vi "Launch Client LNA.vi"(8 "error in (no error)":errorcluster, 11 "Client Controller in":refnum<class "Client Controller.lvclass">) -> (0 "error out":errorcluster, 3 "Client Controller out":refnum<class "Client Controller.lvclass">)   [LabVIEW 2016, in "Client Controller.lvlib" / "Client Controller.lvclass"]
uses:
  Client Controller.lvclass
  C:/Program Files (x86)/National Instruments/LabVIEW 2016/vi.lib/ActorFramework/Actor/Actor.lvclass
  Client LNA/Client LNA.lvclass
  C:/Program Files (x86)/National Instruments/LabVIEW 2016/vi.lib/NI/Actors/Linked Network Actor/Linked Network Actor/Linked Network Actor.lvclass
  <vilib>/ActorFramework/Actor/Actor.lvclass/Actor.ctl
  <vilib>/ActorFramework/Message Enqueuer/Message Enqueuer.lvclass/Message Enqueuer.ctl
  Client Controller.lvclass/Client Controller.ctl
  <vilib>/NI/Actors/Linked Network Actor/Linked Network Actor/Linked Network Actor.lvclass/Linked Network Actor.ctl
  <vilib>/ActorFramework/Message Enqueuer/Init from Existing Queue.vi
  Accessor/Write LNA Active.vi
  <vilib>/ActorFramework/Message Enqueuer/Enqueue.vi
  Messages/Client LNA Started Msg/Client LNA Started Msg.lvclass
  C:/Program Files (x86)/National Instruments/LabVIEW 2016/vi.lib/ActorFramework/Message/Message.lvclass
  <vilib>/ActorFramework/Message Priority Queue/Priority Enqueue.vi
  <vilib>/ActorFramework/Message Enqueuer/Message Enqueuer.lvclass
  <vilib>/NI/Actors/Linked Network Actor/Linked Network Actor/Linked Network Actor.lvclass
  <vilib>/ActorFramework/Actor/Actor.lvclass
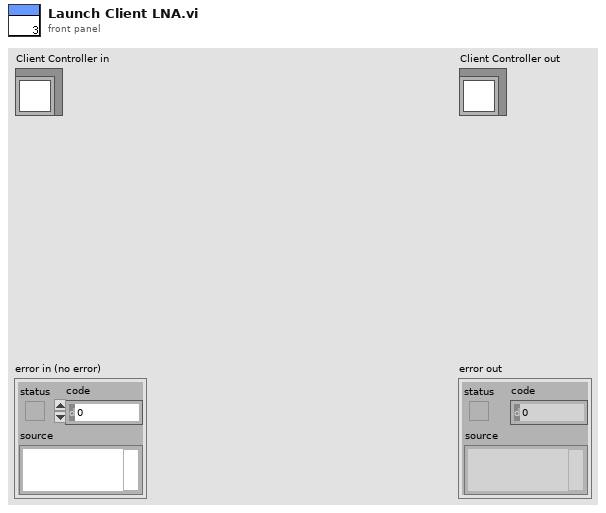
[diagram p1: front panel]
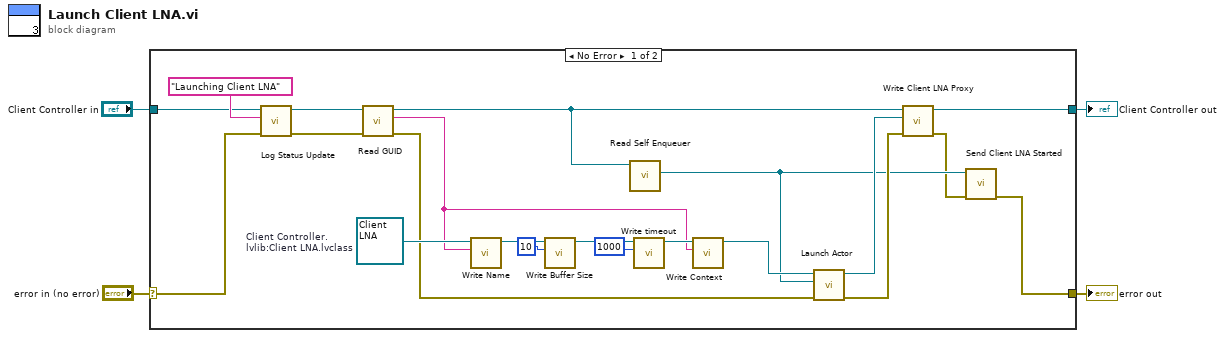
[diagram p0: block diagram]
diagram:
  n1 = case shown="No Error" "error in (no error)" {
    selector: "error in (no error)" -> [w10 w27]
    tunnel: [w5 w27] -> w3
    tunnel: [w20 w26] -> w2
    tunnel: "Client Controller in" -> [w12 w26]
    frame No Error {
      w21 = refnum<class "Client LNA.lvclass"> refnum  # Client Controller.lvlib:Client LNA.lvclass
      n2 = call-dynamic "Log Status Update.vi"("error in (no error)"=w10, "String"="Launching Client LNA", "Controller in"=w12) -> ("error out"=w9:errorcluster, "Controller out"=w11:refnum<class "Client Controller.lvclass">)  [unwired: 7 in]
      n3 = call "Read GUID.vi"("error in (no error)"=w9, "Client Controller in"=w11) -> ("error out"=w17:errorcluster, "GUID"=w16:string, "Client Controller out"=w8:refnum<class "Client Controller.lvclass">)  [unwired: 7 in]
      n4 = call <vilib>:"Write Name.vi"("Name"=w16, "Network Actor in"=w21) -> ("Network Actor out"=w25:refnum<class "Client LNA.lvclass">)  [unwired: 9 in]
      n5 = call <vilib>:"Write Buffer Size.vi"("Buffer Size"=10, "Network Actor in"=w25) -> ("Network Actor out"=w24:refnum<class "Client LNA.lvclass">)  [unwired: 9 in]
      n6 = call <vilib>:"Read Self Enqueuer.vi"("Actor"=w8) -> ("Self Enqueuer"=w7:refnum<class "Message Enqueuer.lvclass">)  [unwired: 10 in]
      n7 = call <vilib>:"Write timeout.vi"("timeout"=1000, "Network Actor in"=w24) -> ("Network Actor out"=w19:refnum<class "Client LNA.lvclass">)  [unwired: 9 in]
      n8 = call <vilib>:"Write Context.vi"("Context"=w16, "Linked Network Actor in"=w19) -> ("Linked Network Actor out"=w18:refnum<class "Client LNA.lvclass">)  [unwired: 9 in]
      n9 = call <vilib>:"Launch Actor.vi"("error in (no error)"=w17, "Actor-to-Caller Enqueuer"=w7, "Actor"=w18) -> ("error out"=w14:errorcluster, "Caller-To-Actor Enqueuer"=w13:refnum<class "Message Enqueuer.lvclass">)  [unwired: 7 in]
      n10 = call "Write Client LNA Proxy.vi"("error in (no error)"=w14, "Actor Framework:Message Enqueuer"=w13, "Client Controller in"=w8) -> ("error out"=w6:errorcluster, "Client Controller out"=w20:refnum<class "Client Controller.lvclass">)  [unwired: 7 in]
      n11 = call "Send Client LNA Started.vi"("error in (no error)"=w6, "Message Enqueuer"=w7) -> ("error out"=w5:errorcluster)  [unwired: 8 in, 1 out]
    }
    frame Error {
    }
  }
  "error out" <- w3
  "Client Controller out" <- w2
